vi "asAcq_dataWait_timeStamp.vi"(0 "reference":refnum<class "OSA.lvclass">, 2 "ms wait":i32, 5 "error in (no error)":errorcluster) -> (14 "duplicate reference":refnum<class "OSA.lvclass">, 18 "dataType":T1[](array[typedef]), 19 "error out":errorcluster)   [LabVIEW 2010, in "OSA.lvclass"]
doc: "Waits for new data to be available.\n\nWhen the datatype array indicator is set to either interferogram or spectrum; data can be read into either a labview- or trace buffer with the dataAcq_get vis.\n\nThe datatype indicator might contain more than one item, (interferogram and spectrum).\n\nSee the acquisition and trace examples for more information."
uses:
  OSA.lvclass
  typeDef/acq_dataType.ctl
  OSA20X_misc.lvlib
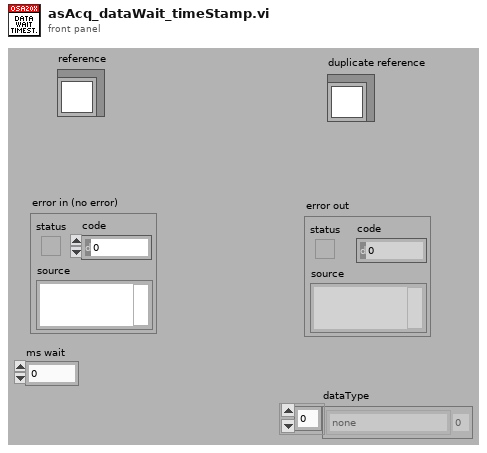
[diagram p1: front panel]
types:
  T1 = typedef "OSA.lvclass/acq_dataType.ctl" = enum16{"none", "interferogram", "spectrum"}
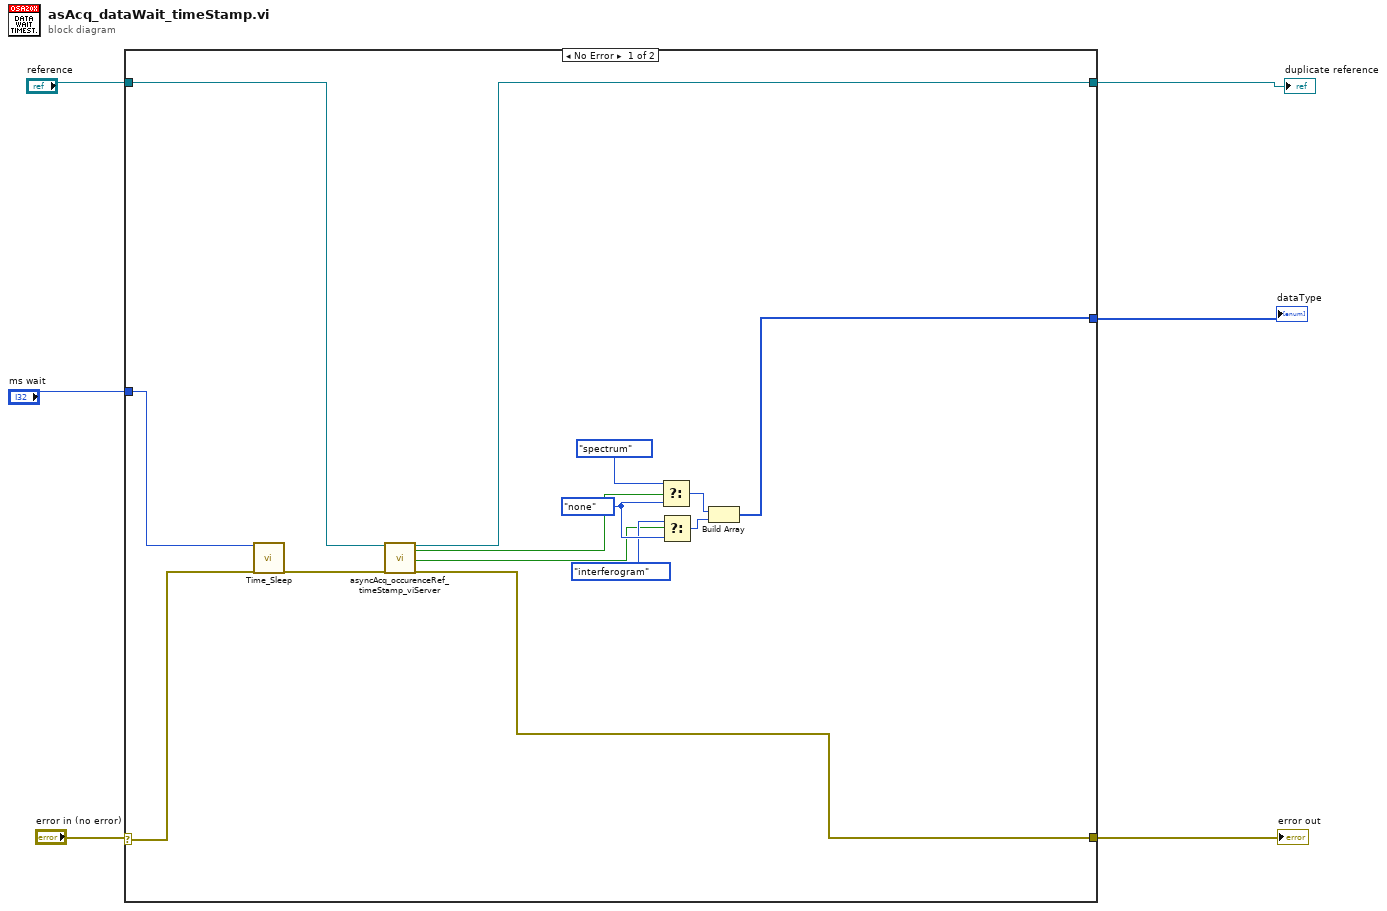
[diagram p0: block diagram]
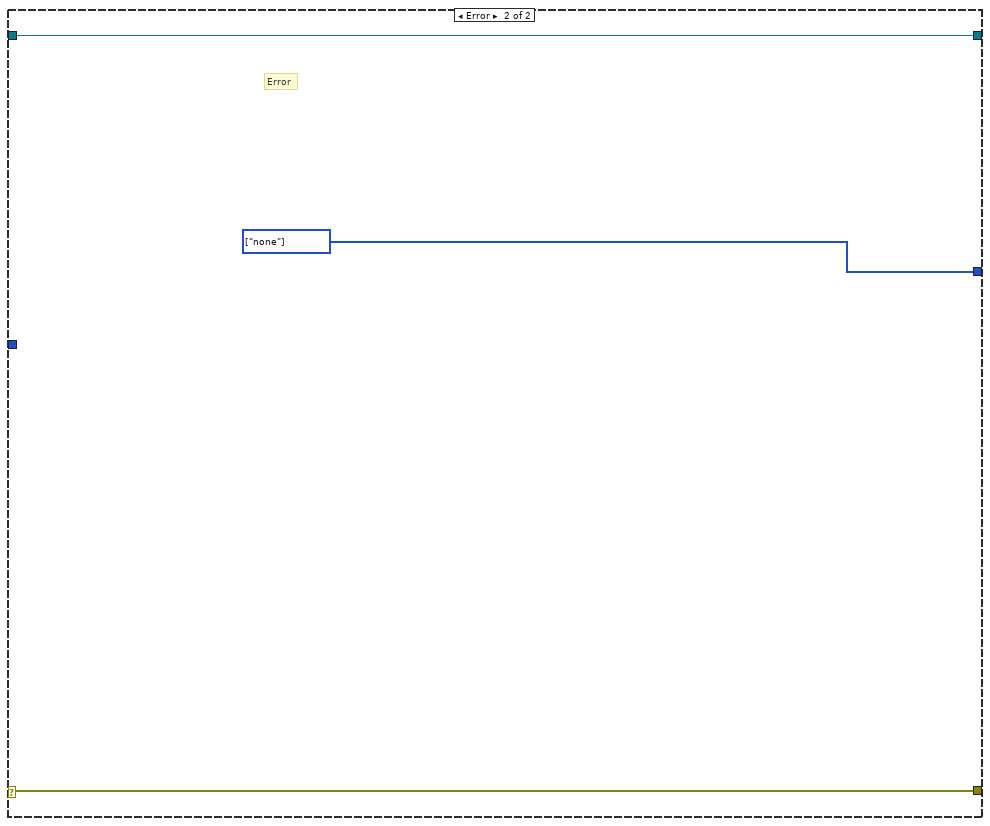
[diagram p2: hidden frame]
diagram:
  n1 = case shown="No Error" "error in (no error)" {
    selector: "error in (no error)" -> [w14 w22]
    tunnel: [w7 w22] -> w6
    tunnel: "reference" -> [w11 w23]
    tunnel: [w8 w23] -> w3
    tunnel: "ms wait" -> [w13 _]
    tunnel: [w15 w21] -> w1
    frame No Error {
      w20 = acq_dataType."none" ("dataType")
      n2 = call "Time_Sleep.vi"("Delay (msec)"=w13, "error in (no error)"=w14) -> ("error out"=w12:errorcluster)  [unwired: 17 in]
      n3 = call "asyncAcq_occurenceRef_timeStamp_viServer.vi"("reference"=w11, "error in (no error)"=w12) -> ("reference out"=w8:refnum<class "OSA.lvclass">, "new spectrum"=w10:bool, "new interferogram"=w9:bool, "error out"=w7:errorcluster)  [unwired: 14 in]
      n4 = Select(t=acq_dataType."spectrum" ("dataType"), s=w10, f=w20) -> (s? t:f=w17:T1)
      n5 = Select(t=acq_dataType."interferogram", s=w9, f=w20) -> (s? t:f=w16:T1)
      n6 = Build Array(w17, w16) -> (w15:T1[])
    }
    frame Error {
      w21 = T1[] [enum."none"] items=["none", "interferogram", "spectrum"] ("appended array")
      # "Error"
    }
  }
  "error out" <- w6
  "duplicate reference" <- w3
  "dataType" <- w1
